vi "Create_Log_CSV_PID2.vi"() -> (3 "path":path)   [LabVIEW 2015]
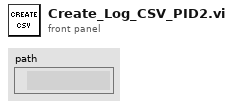
[diagram p1: front panel]
types:
  T1 = enum16{"open", "replace", "create", "open or create", "replace or create", "replace or create with confirmation"}
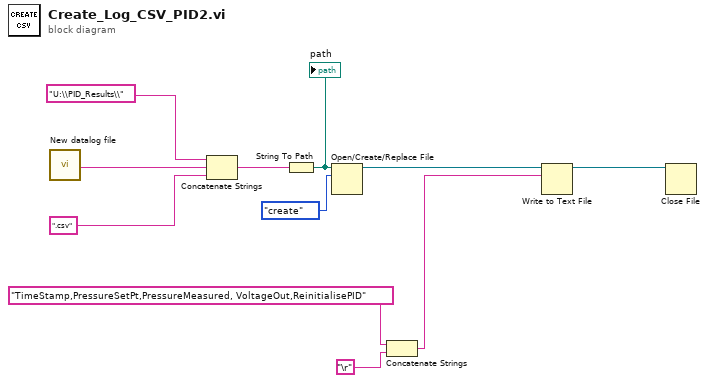
[diagram p0: block diagram]
diagram:
  n1 = call "New datalog file"() -> ("Run Name"=w7:string)  [unwired: 17 in, 2 out]
  n2 = Concatenate Strings("U:\\PID_Results\\", w7, ".csv") -> (w11:string)
  n3 = String To Path(string=w11) -> (path=w8:path)
  "path" <- w8
  n4 = Open/Create/Replace File(file path (use dialog)=w8, operation (0:open)=T1."create") -> (refnum out=w2:refnum<file>)  [unwired: 4 in, 2 out]
  n5 = Concatenate Strings("TimeStamp,PressureSetPt,PressureMeasured, VoltageOut,ReinitialisePID", "\r") -> (w3:string)
  n6 = Write to Text File(file (use dialog)=w2, text=w3) -> (refnum out=w1:refnum<file>)  [unwired: 2 in, 2 out]
  n7 = Close File(refnum=w1) -> ()  [unwired: 1 in, 2 out]
